vi "Example(1).vi"() -> ()   [LabVIEW 2015]
uses:
  Implementations/Ellipse/Ellipse.lvclass
  Implementations/Rectangle/Rectangle.lvclass
  Implementations/Line/Line.lvclass
  Implementations/8 Points Border/8 Points Border.lvclass
  Implementations/2 Points Border/2 Points Border.lvclass
  Interfaces/Shape/Shape.lvclass/Shape.ctl
  Interfaces/Shape/Shape.lvclass
panel:
  out "Border Picture":picture
  in  "Stop Button":bool
  out "Shape Picture":picture
  # "NOTICE -- YOU MUST LEAVE THIS NOTICE IN PLACE.\n\nCopyright (c) 2017, LIANG LIU Shawn.Liu.cn@gmail.com\nAll rights reserved.\n\nRedistribution and use in source and binary forms, with or without modification, are permitted provided that the following conditions are met:\n-Redistributions of source code must retain the above copyright notice, this list of conditions and the following disclaimer.\n-Redistributions in binary form must reproduce the above copyright notice, this list of conditions and the following disclaimer in the documentation and/or other materials provided with the distribution.\n-Neither the name of the eLp nor the names of its contributors may be used to endorse or promote products derived from this software without specific prior written permission.\n\nTHIS SOFTWARE IS PROVIDED BY THE COPYRIGHT HOLDERS AND CONTRIBUTORS \"AS IS\" AND ANY EXPRESS OR IMPLIED WARRANTIES, INCLUDING, BUT NOT LIMITED TO, THE IMPLIED WARRANTIES OF MERCHANTABILITY AND FITNESS FOR A PARTICULAR PURPOSE ARE DISCLAIMED. IN NO EVENT SHALL THE COPYRIGHT HOLDER OR CONTRIBUTORS BE LIABLE FOR ANY DIRECT, INDIRECT, INCIDENTAL, SPECIAL, EXEMPLARY, OR CONSEQUENTIAL DAMAGES (INCLUDING, BUT NOT LIMITED TO, PROCUREMENT OF SUBSTITUTE GOODS OR SERVICES; LOSS OF USE, DATA, OR PROFITS; OR BUSINESS INTERRUPTION) HOWEVER CAUSED AND ON ANY THEORY OF LIABILITY, WHETHER IN CONTRACT, STRICT LIABILITY, OR TORT (INCLUDING NEGLIGENCE OR OTHERWISE) ARISING IN ANY WAY OUT OF THE USE OF THIS SOFTWARE, EVEN IF ADVISED OF THE POSSIBILITY OF SUCH DAMAGE."
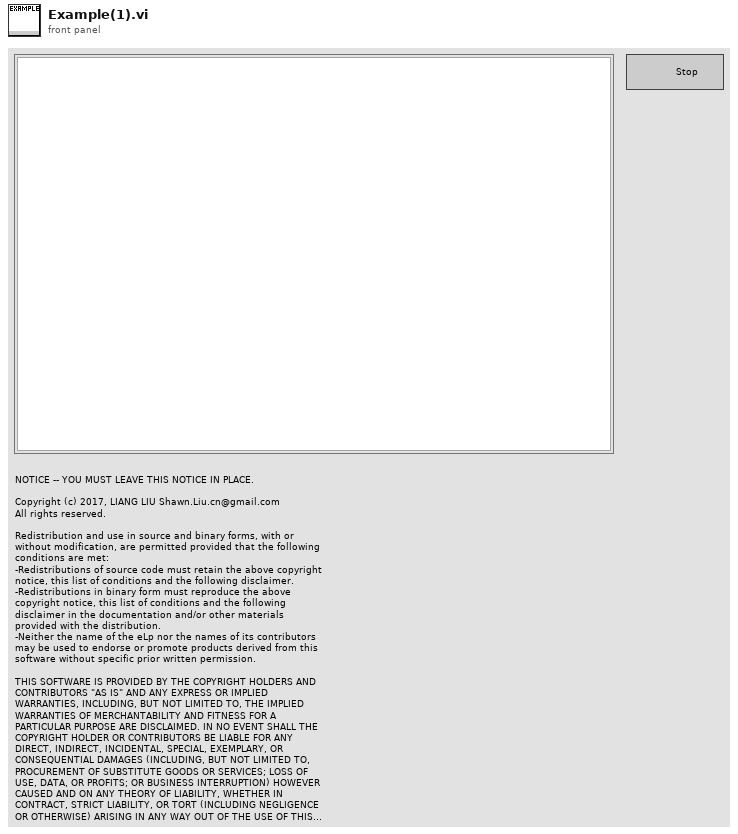
[diagram p1: front panel]
types:
  T1 = typedef "LVPositionTypeDef.ctl" = cluster{"Left":i32, "Top":i32}
  T2 = typedef "LVPoint32TypeDef.ctl" = cluster{"Horizontal":i32, "Vertical":i32}
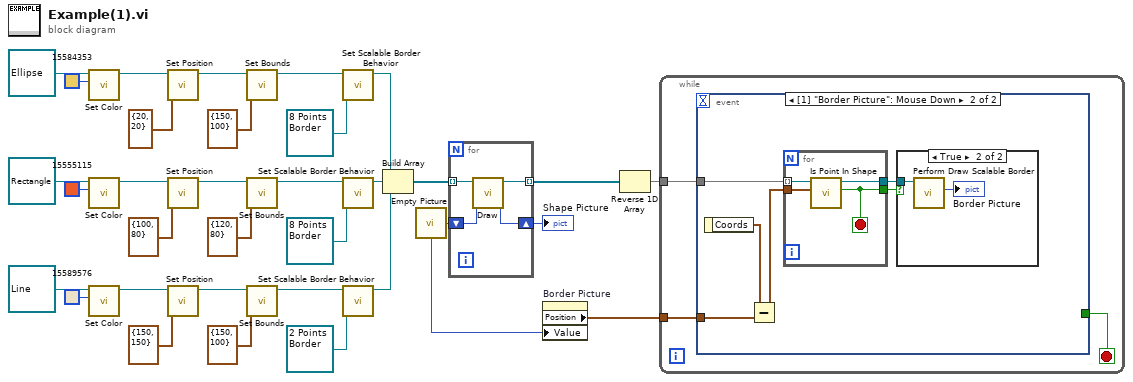
[diagram p0: block diagram]
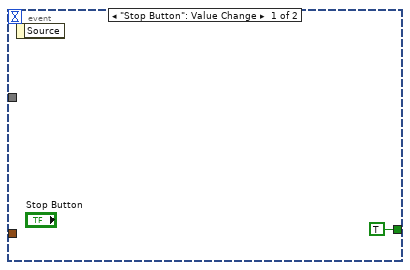
[diagram p2: hidden frame]
diagram:
  n1 = call "Set Color.vi"("Color"=u32 15584353, "Shape in"=refnum<class "Ellipse.lvclass"> refnum ("Ellipse.lvclass")) -> ("Shape out"=w32:refnum<class "Ellipse.lvclass">)  [unwired: 9 in]
  n2 = call "Set Color.vi"("Color"=u32 15555115, "Shape in"=refnum<class "Rectangle.lvclass"> refnum ("Rectangle.lvclass")) -> ("Shape out"=w29:refnum<class "Rectangle.lvclass">)  [unwired: 9 in]
  n3 = call "Set Color.vi"("Color"=u32 15589576, "Shape in"=refnum<class "Line.lvclass"> refnum ("Line.lvclass")) -> ("Shape out"=w9:refnum<class "Line.lvclass">)  [unwired: 9 in]
  n4 = call "Set Position.vi"("Position"=cluster{"Left":i32, "Top":i32} {"Left"=20, "Top"=20}, "Shape in"=w32) -> ("Shape out"=w31:refnum<class "Ellipse.lvclass">)  [unwired: 9 in]
  n5 = call "Set Position.vi"("Position"=cluster{"Left":i32, "Top":i32} {"Left"=100, "Top"=80}, "Shape in"=w29) -> ("Shape out"=w30:refnum<class "Rectangle.lvclass">)  [unwired: 9 in]
  n6 = call "Set Position.vi"("Position"=cluster{"Left":i32, "Top":i32} {"Left"=150, "Top"=150}, "Shape in"=w9) -> ("Shape out"=w8:refnum<class "Line.lvclass">)  [unwired: 9 in]
  n7 = call "Set Bounds.vi"("Bounds"=cluster{"Width":u32, "Height":u32} {"Width"=150, "Height"=100}, "Shape in"=w31) -> ("Shape out"=w14:refnum<class "Ellipse.lvclass">)  [unwired: 9 in]
  n8 = call "Set Bounds.vi"("Bounds"=cluster{"Width":u32, "Height":u32} {"Width"=120, "Height"=80}, "Shape in"=w30) -> ("Shape out"=w25:refnum<class "Rectangle.lvclass">)  [unwired: 9 in]
  n9 = call "Set Bounds.vi"("Bounds"=cluster{"Width":u32, "Height":u32} {"Width"=150, "Height"=100}, "Shape in"=w8) -> ("Shape out"=w7:refnum<class "Line.lvclass">)  [unwired: 9 in]
  n10 = call "Set Scalable Border Behavior.vi"("Scalable Border Behavior"=refnum<class "8 Points Border.lvclass"> refnum ("8 Points Border.lvclass"), "Shape in"=w14) -> ("Shape out"=w6:refnum<class "Ellipse.lvclass">)  [unwired: 9 in]
  n11 = call "Set Scalable Border Behavior.vi"("Scalable Border Behavior"=refnum<class "8 Points Border.lvclass"> refnum ("8 Points Border.lvclass"), "Shape in"=w25) -> ("Shape out"=w5:refnum<class "Rectangle.lvclass">)  [unwired: 9 in]
  n12 = call "Set Scalable Border Behavior.vi"("Scalable Border Behavior"=refnum<class "2 Points Border.lvclass"> refnum ("2 Points Border.lvclass"), "Shape in"=w7) -> ("Shape out"=w4:refnum<class "Line.lvclass">)  [unwired: 9 in]
  n13 = Build Array(w6, w5, w4) -> (w24:refnum<class "Shape.lvclass">[])
  n14 = call "Empty Picture"() -> ("empty picture"=w16:picture)
  n15 = for {
    tunnel: w24 -> [w37] mode=indexing
    shift-right: [w36] -> w23
    shift-left: w16 -> [w35]
    tunnel: [w34] -> w18 mode=indexing
    n16 = call-dynamic "Draw.vi"("Picture in"=w35, "Shape in"=w37) -> ("Picture out"=w36:picture, "Shape out"=w34:refnum<class "Shape.lvclass">)  [unwired: 7 in, 1 out]
  }
  "Shape Picture" <- w23
  n17 = property on="Border Picture" class="Pict"("Value"=w16) -> ("Position"=w15:T1)  [unwired: 2 in, 2 out]
  n18 = Reverse 1D Array(array=w18) -> (reversed array=w17:refnum<class "Shape.lvclass">[])
  n19 = while {
    tunnel: w17 -> [w40]
    tunnel: w15 -> [w38]
    stop <- w39 stop-if-true
    n20 = event shown="[1] \"Border Picture\": Mouse Down" {
      selector: _ -> [_ _]
      dyn-events: _ -> [_ _]
      timeout: _ -> [_ _]
      tunnel: w40 -> [_ w47]
      tunnel: [TRUE _] -> w39
      tunnel: w38 -> [_ w44]
      event "Stop Button": Value Change {
        n21 = event-data() -> ()  [unwired: 1 in, 1 out]
      }
      event "Border Picture": Mouse Down {
        n22 = event-data() -> ("Coords"=w43:T2)  [unwired: 1 in]
        n23 = Subtract(x=w43, y=w44) -> (x-y=w42:T2)
        n24 = for {
          tunnel: w47 -> [w53] mode=indexing
          tunnel: [w52] -> w46
          tunnel: [w51] -> w45
          tunnel: w42 -> [w50]
          stop <- w52 stop-if-true
          n25 = call-dynamic "Is Point In Shape.vi"("Point"=w50, "Shape in"=w53) -> ("Point In Shape?"=w52:bool, "Shape out"=w51:refnum<class "Shape.lvclass">)  [unwired: 7 in, 1 out]
        }
        n26 = case shown="True" w46 {
          tunnel: w45 -> [_ w49]
          frame False {
          }
          frame True {
            n27 = call-dynamic "Perform Draw Scalable Border.vi"("Shape in"=w49) -> ("Border out"=→"Border Picture":picture)  [unwired: 8 in, 2 out]
          }
        }
      }
    }
  }
